vi "replace cursor - plot ref - V4.vi"(0 "plot ref IN":refnum<vi>, 1 "new X":dbl=nan, 3 "new  Y":dbl=nan, 4 "window IN":T2={"window y"=0.0021014740628288917, "center x"=44850.89441339177, "center y"=2.5658109925320947, "window x"=17480.201988350764} {"window x" format="%#9_9f"; "center y" format="%#9_9f"; "center x" format="%#9_9f"}, 5 "cursor index":i32, 6 "cursor action":T3=enum."write", 7 "label":enum16{"hide", "show x", "show y", "show (x,y)"}(ring), 9 "x-label":string, 11 "y-label":string, 12 "Color Box":u32(colorbox)=327424, 13 "cursor state":T4=enum."boring") -> (14 "plot ref OUT":refnum<vi>, 15 "read X":dbl, 18 "read Y":dbl, 19 "2Dwindow bounds out":T1={"min y"=0.0021014740628288917, "max x"=44850.89441339177, "min x"=2.5658109925320947, "max y"=17480.201988350764} {"max y" format="%#9_9f"; "min x" format="%#9_9f"; "max x" format="%#9_9f"})   [LabVIEW 2021]
uses:
  cursor sate.ctl
  cursor action.ctl
  2Dwindow-centerwin.ctl
  2Dwindow-bounds.ctl
  stack action -- control.ctl
  range multiplier action.ctl
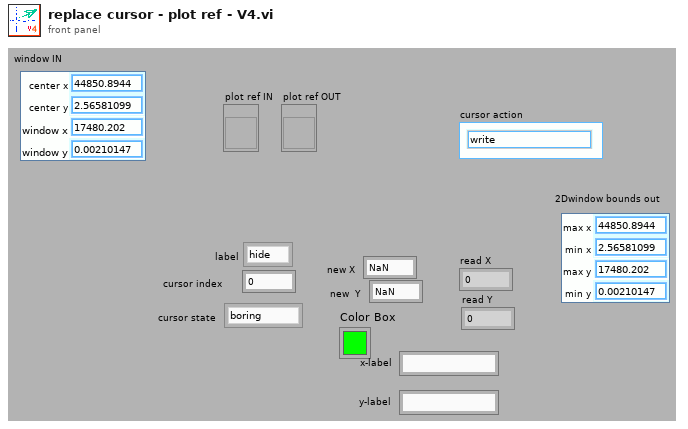
[diagram p1: front panel]
types:
  T1 = typedef "2Dwindow-bounds.ctl" = cluster{"min y":dbl, "max x":dbl, "min x":dbl, "max y":dbl}
  T2 = typedef "2Dwindow-centerwin.ctl" = cluster{"window y":dbl, "center x":dbl, "center y":dbl, "window x":dbl}
  T3 = typedef "cursor action.ctl" = enum16{"range", "read", "write", "check", "zoom out", "smart zoom out", "zoom to aspect ratio 1", "zoom to win", "zoom out 20%", "zoom in 20%", "-empty", "smart zoom out&aspect", "move range left 20%", "move range right 20%", "move range up 20%", "move range down 20%", "zoom to X win", "zoom to Y win", "zoom out X", "zoom out Y", "zoom in X", "zoom in Y", "check plot scale", "set plot color", "set Xlabel", "set Ylabel", "set cursor color", "setlength", "empty", "hide plot", "unhide plot", "checklngth", "extend +1 if short", "extend +n if short"}
  T4 = typedef "cursor sate.ctl" = enum16{"normal", "alert", "fuzzy", "interesting", "boring", "colored"}
  T5 = typedef "stack action -- control.ctl" = enum16{"push", "pop", "check", "init"}
  T6 = typedef "LVCursorListTypeDef.ctl" = cluster{"Name":string, "Color":u32, "Style":u8, "Point Style":u8, "Name Visible":bool, "Allow Drag":bool, "Cursor Mode":u32, "Plot":i32, "Index":i32, "Position":cluster{"X":dbl, "Y":dbl}, "X Scale":u32, "Y Scale":u32, "Watch Plots":i32[], "Watch All Plots":bool, "Plot Area":i32, "Label Offset":cluster{"X":dbl, "Y":dbl}}[]
  T7 = typedef "range multiplier action.ctl" = enum16{"shift", "zoom", "check"}
  T8 = cluster{"Name":string, "Color":u32, "Style":u8, "Point Style":u8, "Name Visible":bool, "Allow Drag":bool, "Cursor Mode":u32, "Plot":i32, "Index":i32, "Position":cluster{"X":dbl, "Y":dbl}, "X Scale":u32, "Y Scale":u32, "Watch Plots":i32[], "Watch All Plots":bool, "Plot Area":i32, "Label Offset":cluster{"X":dbl, "Y":dbl}}
  T9 = typedef "LVRangeTypeDef.ctl" = cluster{"Minimum":dbl, "Maximum":dbl, "Increment":dbl, "Minor Increment":dbl, "Start":dbl}
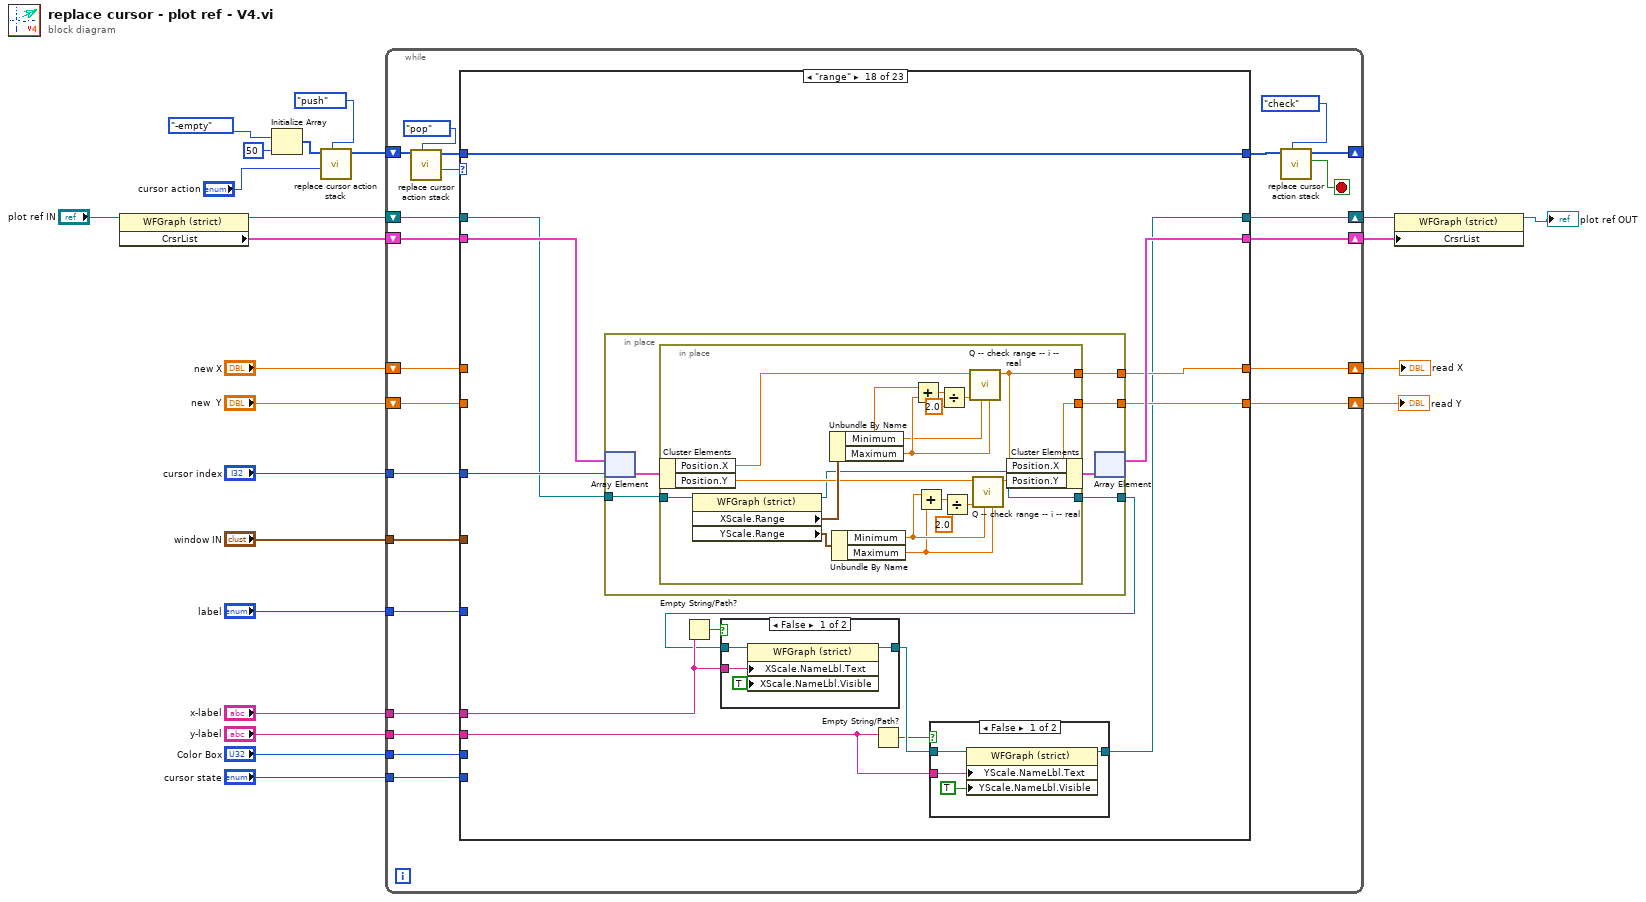
[diagram p0: block diagram]
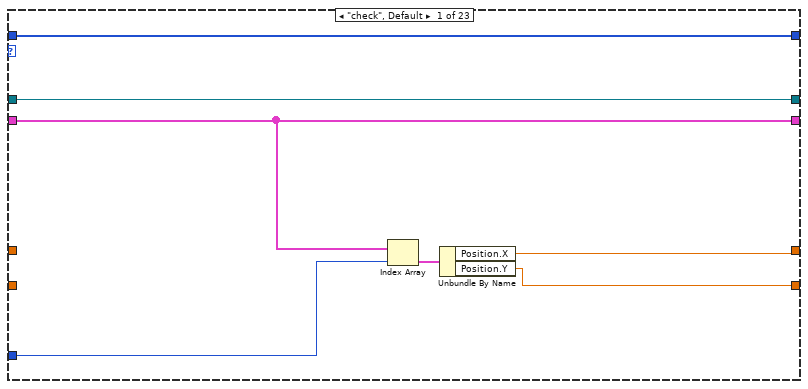
[diagram p2: hidden frame]
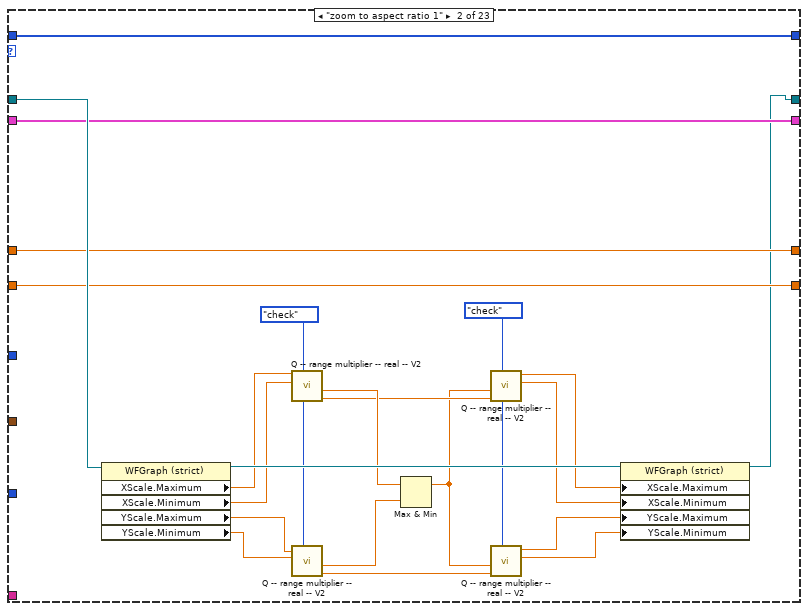
[diagram p3: hidden frame]
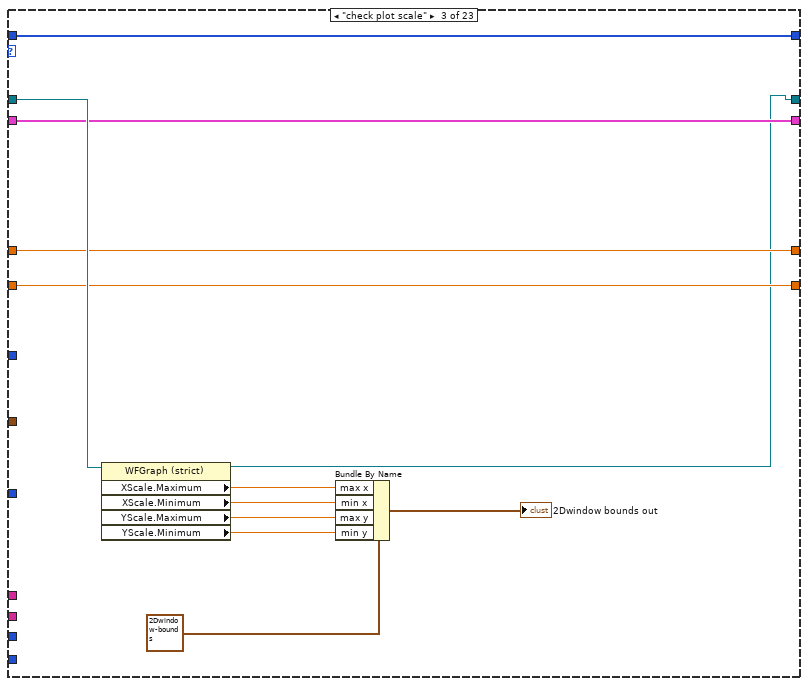
[diagram p4: hidden frame]
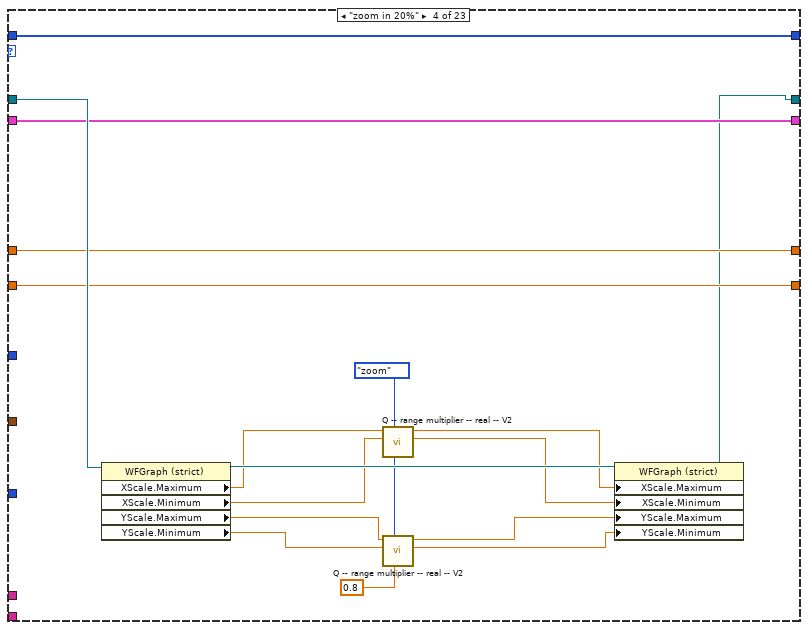
[diagram p5: hidden frame]
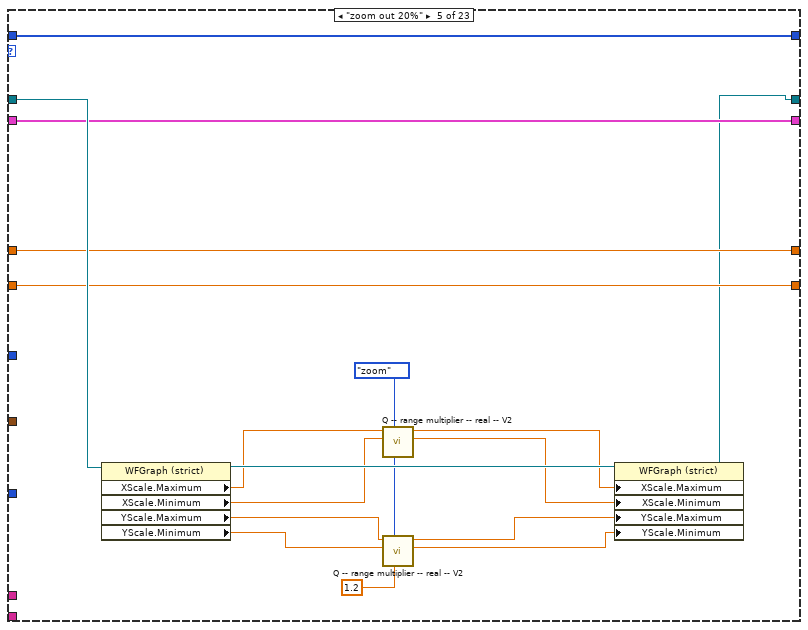
[diagram p6: hidden frame]
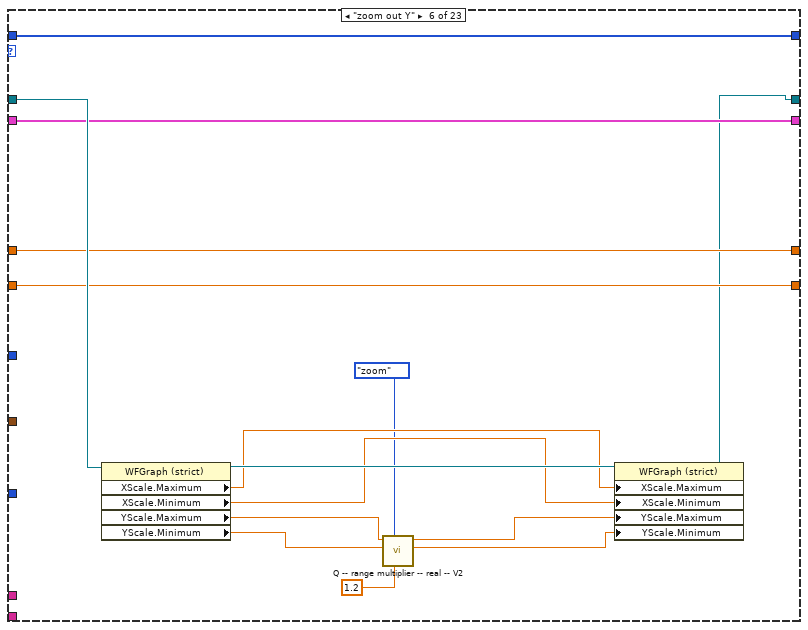
[diagram p7: hidden frame]
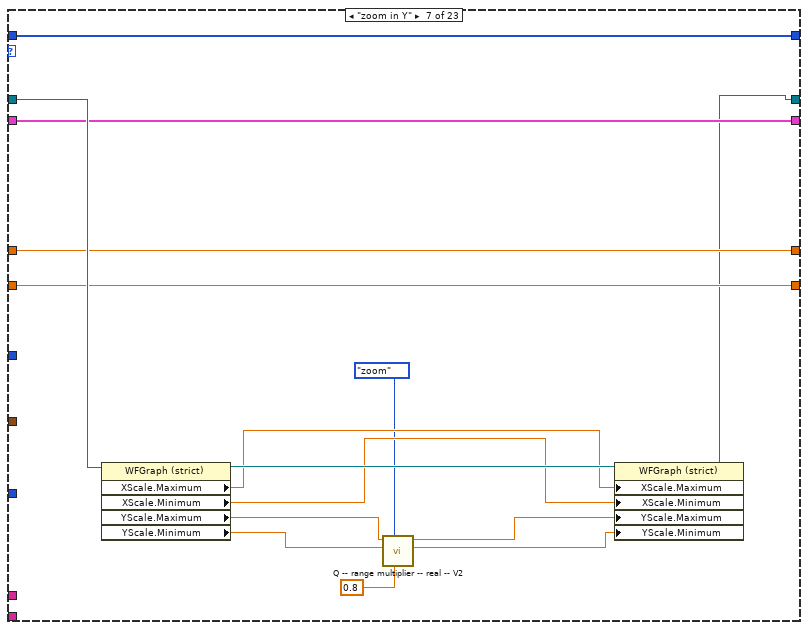
[diagram p8: hidden frame]
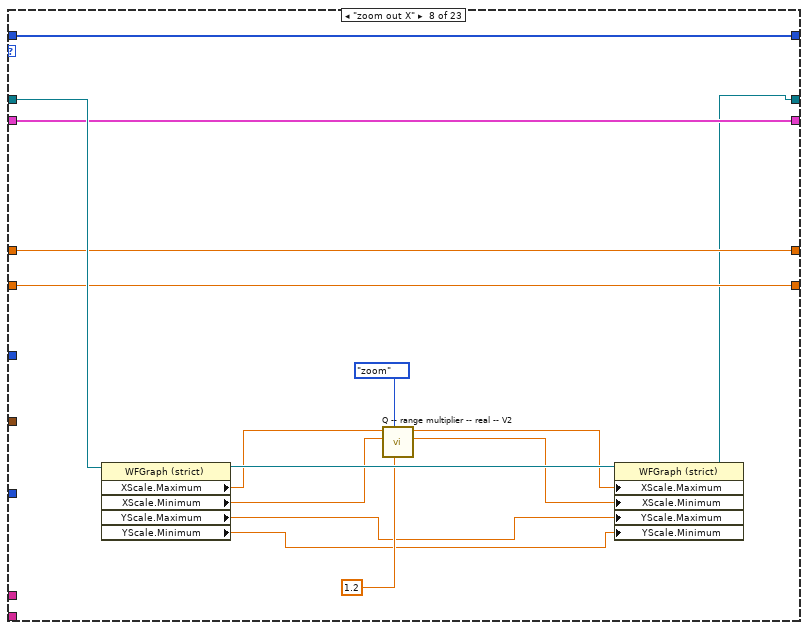
[diagram p9: hidden frame]
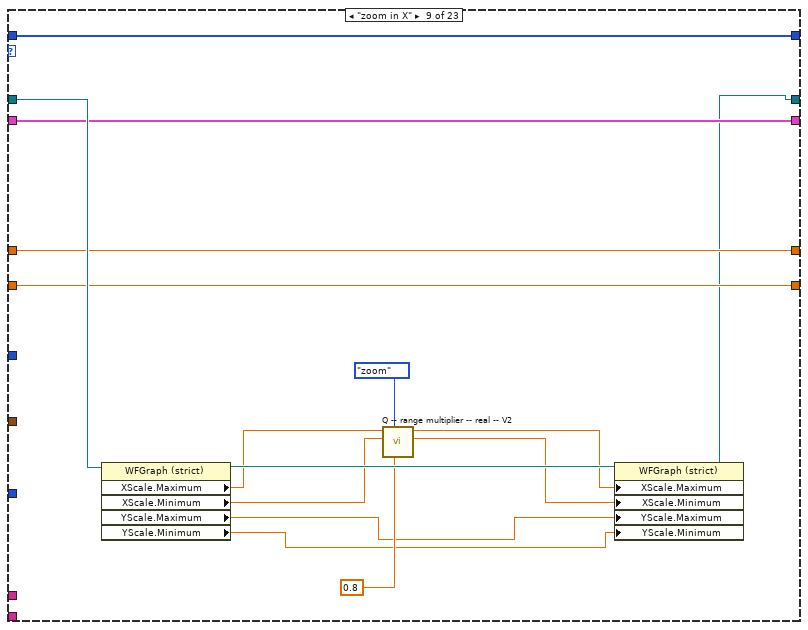
[diagram p10: hidden frame]
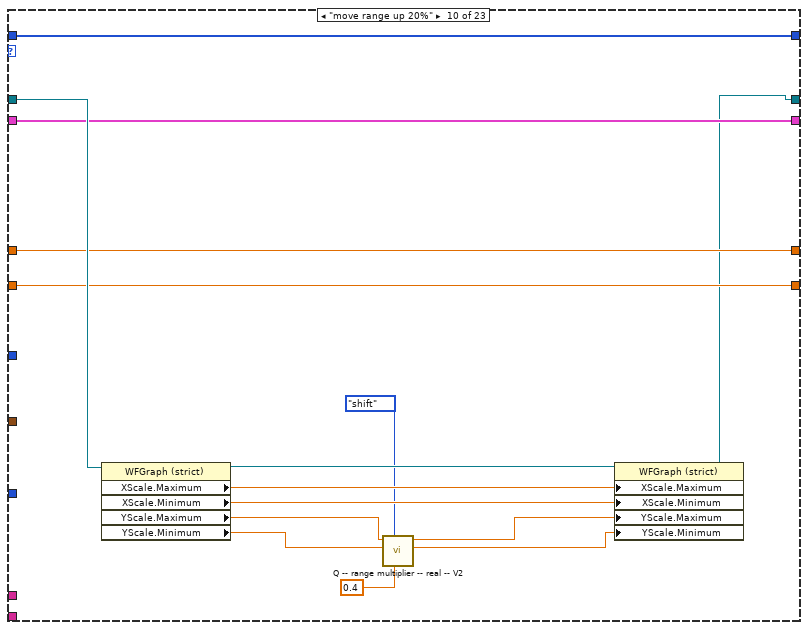
[diagram p11: hidden frame]
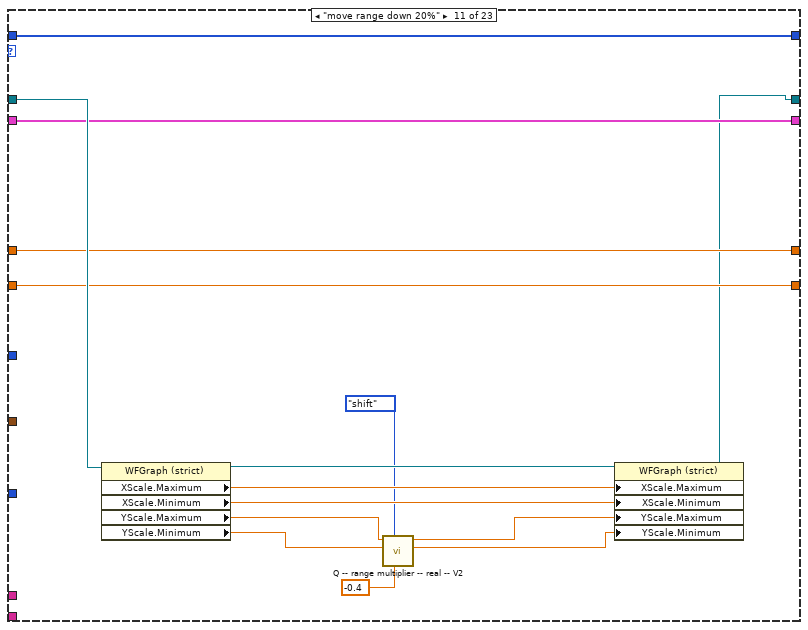
[diagram p12: hidden frame]
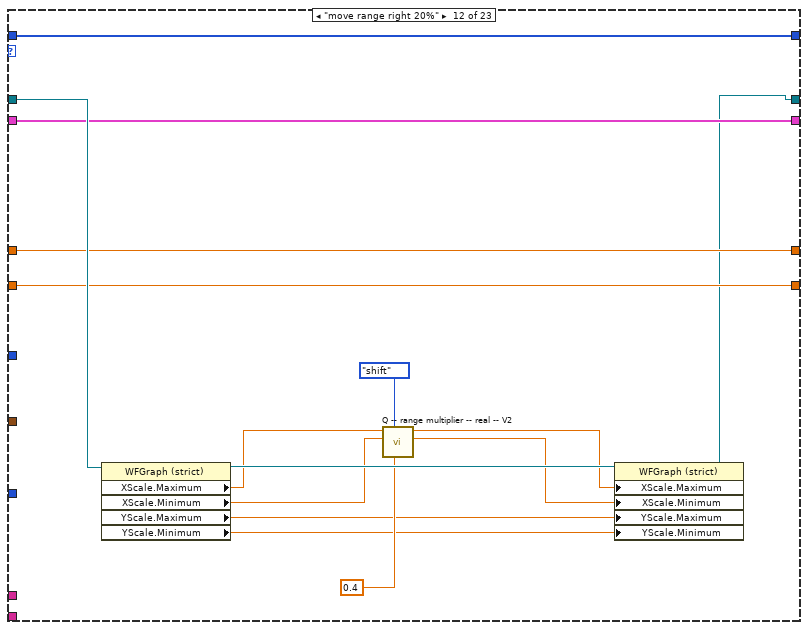
[diagram p13: hidden frame]
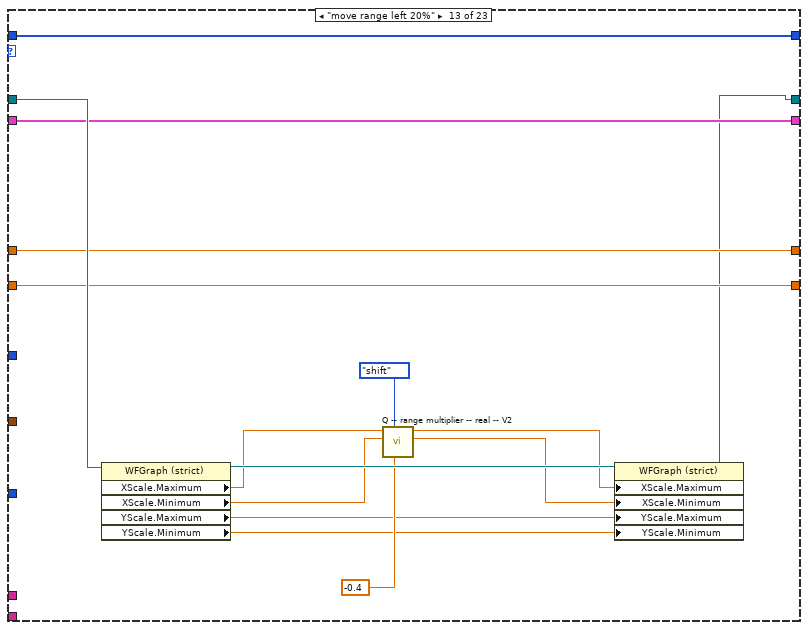
[diagram p14: hidden frame]
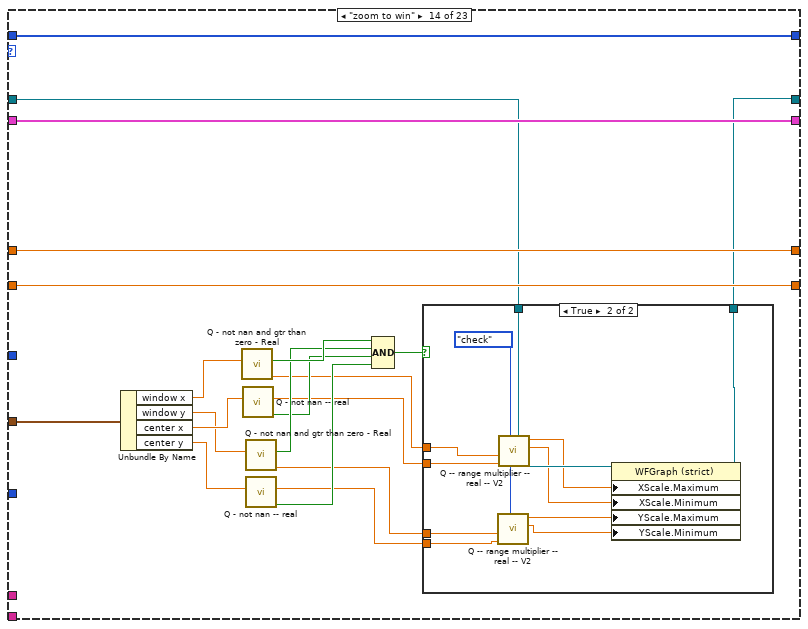
[diagram p15: hidden frame]
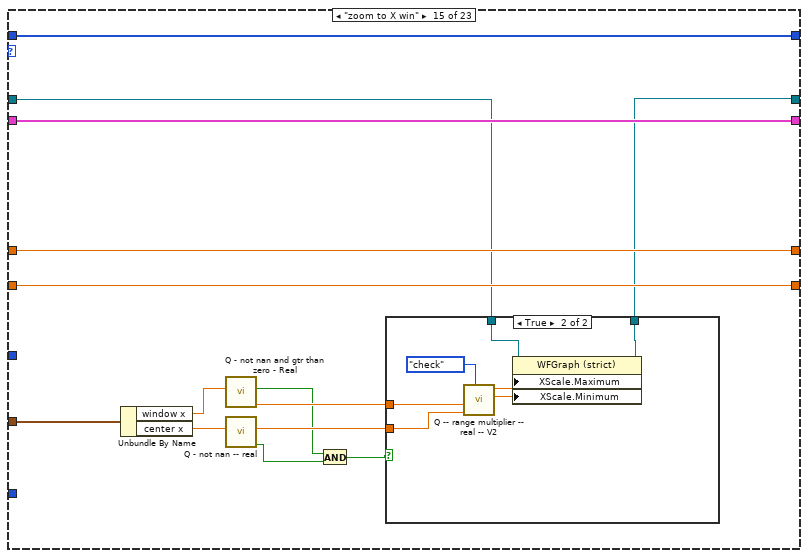
[diagram p17: hidden frame]
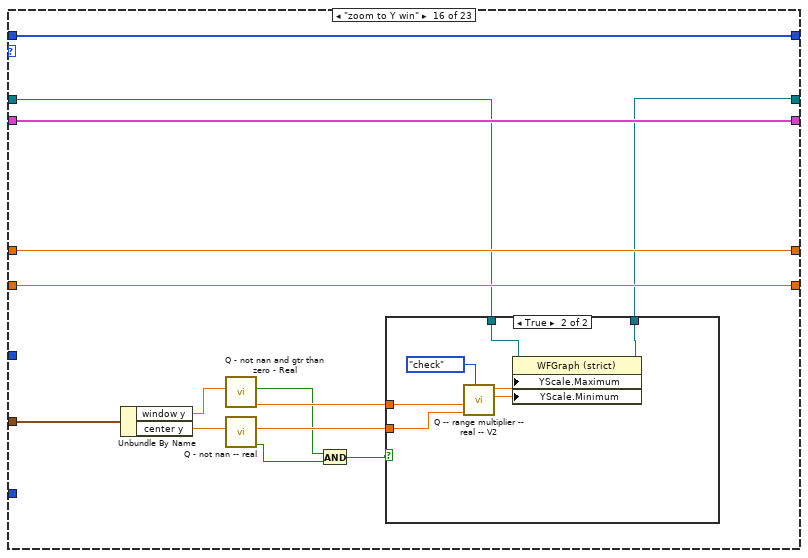
[diagram p19: hidden frame]
diagram:
  n1 = property on="Property Node" class="WFGraph (strict)"(reference="plot ref IN") -> (reference out=w15:refnum<vi>, "CrsrList"=w20:T6)  [unwired: 1 in, 1 out]
  n2 = Initialize Array(cursor_action."-empty" ("cursor action"), 50 ("dimension size")) -> (w8:T3[])
  n3 = call "replace cursor action stack.vi"("stack action"=stack_action_--_control."push", "cursor action"="cursor action", "command stack In"=w8) -> ("command stack Out"=w5:T3[])  [unwired: 6 in, 2 out]
  n4 = while {
    tunnel: "cursor index" -> [w46]
    tunnel: "label" -> [w42]
    tunnel: "Color Box" -> [w41]
    tunnel: "cursor state" -> [w40]
    tunnel: "x-label" -> [w37]
    tunnel: "y-label" -> [w36]
    tunnel: "window IN" -> [w34]
    shift-right: [w35] -> w12
    shift-left: w20 -> [w43]
    shift-right: [w39] -> w16
    shift-left: w15 -> [w38]
    shift-right: [w29] -> _
    shift-left: w5 -> [w33]
    shift-right: [w26] -> w3
    shift-left: "new  Y" -> [w45]
    shift-right: [w25] -> w4
    shift-left: "new X" -> [w44]
    stop <- w30 stop-if-true
    n5 = call "replace cursor action stack.vi"("stack action"=stack_action_--_control."pop", "command stack In"=w33) -> ("cursor action Out"=w31:T3, "command stack Out"=w27:T3[])  [unwired: 7 in, 1 out]
    n6 = case shown="\"range\"" w31 {
      tunnel: w46 -> [w51 _ _ _ _ _ _ _ _ _ _ _ _ _ _ _ _ w337 _ _ w453 w462 w507]
      tunnel: w43 -> [w52 w73 w86 w102 w119 w134 w149 w164 w179 w194 w209 w224 w239 w261 w287 w309 w318 w339 w395 w431 w451 w464 w509]
      tunnel: w45 -> [_ w71 w84 w100 w117 w132 w147 w162 w177 w192 w207 w222 w237 w259 w285 w307 w320 _ w390 w426 _ w465 w501]
      tunnel: w44 -> [_ w72 w85 w101 w118 w133 w148 w163 w178 w193 w208 w223 w238 w260 w286 w308 w321 _ w391 w427 _ w466 w502]
      tunnel: [w49 w72 w85 w101 w118 w133 w148 w163 w178 w193 w208 w223 w238 w260 w286 w308 w321 w336 w391 w427 w450 w461 w502] -> w25
      tunnel: [w48 w71 w84 w100 w117 w132 w147 w162 w177 w192 w207 w222 w237 w259 w285 w307 w320 w335 w390 w426 w449 w460 w501] -> w26
      tunnel: w42 -> [_ _ _ _ _ _ _ _ _ _ _ _ _ _ _ _ _ _ _ _ _ w459 w506]
      tunnel: w41 -> [_ _ _ _ _ _ _ _ _ _ _ _ _ _ _ _ _ _ _ _ _ w458 w505]
      tunnel: w40 -> [_ _ _ _ _ _ _ _ _ _ _ _ _ _ _ _ _ _ _ _ _ w457 _]
      tunnel: [w53 w69 w82 w98 w115 w130 w145 w160 w175 w190 w205 w220 w235 w255 w281 w303 w319 w327 w392 w428 w448 w456 w504] -> w39
      tunnel: w38 -> [w53 w74 w87 w103 w120 w135 w150 w165 w180 w195 w210 w225 w240 w257 w283 w305 w319 w334 w394 w430 w448 w456 w504]
      tunnel: w37 -> [_ _ _ _ _ _ _ _ _ _ _ _ _ _ _ _ _ w332 _ _ _ _ _]
      tunnel: w36 -> [_ _ _ _ _ _ _ _ _ _ _ _ _ _ _ _ _ w329 _ _ _ _ _]
      tunnel: [w52 w73 w86 w102 w119 w134 w149 w164 w179 w194 w209 w224 w239 w261 w287 w309 w318 w338 w395 w431 w451 w463 w508] -> w35
      tunnel: w34 -> [_ _ _ _ _ _ _ _ _ _ _ _ _ w258 w284 w306 _ _ _ _ _ _ _]
      tunnel: [w47 w70 w83 w99 w116 w131 w146 w161 w176 w191 w206 w221 w236 w256 w282 w304 w323 w326 w376 w413 w447 w455 w503] -> w28
      tunnel: w27 -> [w47 w70 w83 w99 w116 w131 w146 w161 w176 w191 w206 w221 w236 w256 w282 w304 w324 w326 w376 w413 w447 w455 w503]
      frame "check", Default {
        n7 = Index Array(array=w52, index=w51) -> (element=w50:T8)
        n8 = Unbundle By Name(w50) -> ("Position.X"=w49:dbl, "Position.Y"=w48:dbl)
      }
      frame "zoom to aspect ratio 1" {
        w58 = range_multiplier_action."check" ("rage multiplier action")
        w64 = range_multiplier_action."check" ("rage multiplier action")
        n9 = property on="Property Node" class="WFGraph (strict)"(reference=w74) -> (reference out=w75:refnum<vi>, "XScale.Maximum"=w68:dbl, "XScale.Minimum"=w67:dbl, "YScale.Maximum"=w66:dbl, "YScale.Minimum"=w65:dbl)  [unwired: 1 in, 1 out]
        n10 = call "Q -- range multiplier -- real -- V2.vi"("rage multiplier action"=w64, "lower"=w67, "upper"=w68) -> ("center OUT"=w61:dbl, "window OUT"=w63:dbl)  [unwired: 5 in, 2 out]
        n11 = call "Q -- range multiplier -- real -- V2.vi"("rage multiplier action"=w64, "lower"=w65, "upper"=w66) -> ("center OUT"=w60:dbl, "window OUT"=w62:dbl)  [unwired: 5 in, 2 out]
        n12 = Max & Min(x=w63, y=w62) -> (max(x,y)=w59:dbl)  [unwired: 1 out]
        n13 = call "Q -- range multiplier -- real -- V2.vi"("rage multiplier action"=w58, "center"=w61, "window"=w59) -> ("lower OUT"=w54:dbl, "upper OUT"=w55:dbl)  [unwired: 5 in, 2 out]
        n14 = call "Q -- range multiplier -- real -- V2.vi"("rage multiplier action"=w58, "center"=w60, "window"=w59) -> ("lower OUT"=w56:dbl, "upper OUT"=w57:dbl)  [unwired: 5 in, 2 out]
        n15 = property on="Property Node" class="WFGraph (strict)"(reference=w75, "XScale.Maximum"=w55, "XScale.Minimum"=w54, "YScale.Maximum"=w57, "YScale.Minimum"=w56) -> (reference out=w69:refnum<vi>)  [unwired: 1 in, 1 out]
      }
      frame "check plot scale" {
        n16 = property on="Property Node" class="WFGraph (strict)"(reference=w87) -> (reference out=w82:refnum<vi>, "XScale.Maximum"=w80:dbl, "XScale.Minimum"=w79:dbl, "YScale.Maximum"=w78:dbl, "YScale.Minimum"=w77:dbl)  [unwired: 1 in, 1 out]
        n17 = Bundle By Name(cluster=T1 {"min y"=0.0021014740628288917, "max x"=44850.89441339177, "min x"=2.5658109925320947, "max y"=17480.201988350764} ("2Dwindow bounds out"), "max x"=w80, "min x"=w79, "max y"=w78, "min y"=w77) -> (→"2Dwindow bounds out":T1)
      }
      frame "zoom in 20%" {
        w89 = range_multiplier_action."zoom" ("rage multiplier action")
        w88 = 0.8
        n18 = property on="Property Node" class="WFGraph (strict)"(reference=w103) -> (reference out=w104:refnum<vi>, "XScale.Maximum"=w97:dbl, "XScale.Minimum"=w96:dbl, "YScale.Maximum"=w93:dbl, "YScale.Minimum"=w92:dbl)  [unwired: 1 in, 1 out]
        n19 = call "Q -- range multiplier -- real -- V2.vi"("factor"=w88, "rage multiplier action"=w89, "lower"=w96, "upper"=w97) -> ("lower OUT"=w94:dbl, "upper OUT"=w95:dbl)  [unwired: 4 in, 2 out]
        n20 = call "Q -- range multiplier -- real -- V2.vi"("factor"=w88, "rage multiplier action"=w89, "lower"=w92, "upper"=w93) -> ("lower OUT"=w90:dbl, "upper OUT"=w91:dbl)  [unwired: 4 in, 2 out]
        n21 = property on="Property Node" class="WFGraph (strict)"(reference=w104, "XScale.Maximum"=w95, "XScale.Minimum"=w94, "YScale.Maximum"=w91, "YScale.Minimum"=w90) -> (reference out=w98:refnum<vi>)  [unwired: 1 in, 1 out]
      }
      frame "zoom out 20%" {
        w106 = range_multiplier_action."zoom" ("rage multiplier action")
        w105 = 1.2
        n22 = property on="Property Node" class="WFGraph (strict)"(reference=w120) -> (reference out=w121:refnum<vi>, "XScale.Maximum"=w114:dbl, "XScale.Minimum"=w113:dbl, "YScale.Maximum"=w110:dbl, "YScale.Minimum"=w109:dbl)  [unwired: 1 in, 1 out]
        n23 = call "Q -- range multiplier -- real -- V2.vi"("factor"=w105, "rage multiplier action"=w106, "lower"=w113, "upper"=w114) -> ("lower OUT"=w111:dbl, "upper OUT"=w112:dbl)  [unwired: 4 in, 2 out]
        n24 = call "Q -- range multiplier -- real -- V2.vi"("factor"=w105, "rage multiplier action"=w106, "lower"=w109, "upper"=w110) -> ("lower OUT"=w107:dbl, "upper OUT"=w108:dbl)  [unwired: 4 in, 2 out]
        n25 = property on="Property Node" class="WFGraph (strict)"(reference=w121, "XScale.Maximum"=w112, "XScale.Minimum"=w111, "YScale.Maximum"=w108, "YScale.Minimum"=w107) -> (reference out=w115:refnum<vi>)  [unwired: 1 in, 1 out]
      }
      frame "zoom out Y" {
        n26 = property on="Property Node" class="WFGraph (strict)"(reference=w135) -> (reference out=w136:refnum<vi>, "XScale.Maximum"=w124:dbl, "XScale.Minimum"=w123:dbl, "YScale.Maximum"=w129:dbl, "YScale.Minimum"=w128:dbl)  [unwired: 1 in, 1 out]
        n27 = call "Q -- range multiplier -- real -- V2.vi"("factor"=1.2, "rage multiplier action"=range_multiplier_action."zoom", "lower"=w128, "upper"=w129) -> ("lower OUT"=w126:dbl, "upper OUT"=w127:dbl)  [unwired: 4 in, 2 out]
        n28 = property on="Property Node" class="WFGraph (strict)"(reference=w136, "XScale.Maximum"=w124, "XScale.Minimum"=w123, "YScale.Maximum"=w127, "YScale.Minimum"=w126) -> (reference out=w130:refnum<vi>)  [unwired: 1 in, 1 out]
      }
      frame "zoom in Y" {
        n29 = property on="Property Node" class="WFGraph (strict)"(reference=w150) -> (reference out=w151:refnum<vi>, "XScale.Maximum"=w139:dbl, "XScale.Minimum"=w138:dbl, "YScale.Maximum"=w144:dbl, "YScale.Minimum"=w143:dbl)  [unwired: 1 in, 1 out]
        n30 = call "Q -- range multiplier -- real -- V2.vi"("factor"=0.8, "rage multiplier action"=range_multiplier_action."zoom", "lower"=w143, "upper"=w144) -> ("lower OUT"=w141:dbl, "upper OUT"=w142:dbl)  [unwired: 4 in, 2 out]
        n31 = property on="Property Node" class="WFGraph (strict)"(reference=w151, "XScale.Maximum"=w139, "XScale.Minimum"=w138, "YScale.Maximum"=w142, "YScale.Minimum"=w141) -> (reference out=w145:refnum<vi>)  [unwired: 1 in, 1 out]
      }
      frame "zoom out X" {
        n32 = property on="Property Node" class="WFGraph (strict)"(reference=w165) -> (reference out=w166:refnum<vi>, "XScale.Maximum"=w159:dbl, "XScale.Minimum"=w158:dbl, "YScale.Maximum"=w153:dbl, "YScale.Minimum"=w152:dbl)  [unwired: 1 in, 1 out]
        n33 = call "Q -- range multiplier -- real -- V2.vi"("factor"=1.2, "rage multiplier action"=range_multiplier_action."zoom", "lower"=w158, "upper"=w159) -> ("lower OUT"=w156:dbl, "upper OUT"=w157:dbl)  [unwired: 4 in, 2 out]
        n34 = property on="Property Node" class="WFGraph (strict)"(reference=w166, "XScale.Maximum"=w157, "XScale.Minimum"=w156, "YScale.Maximum"=w153, "YScale.Minimum"=w152) -> (reference out=w160:refnum<vi>)  [unwired: 1 in, 1 out]
      }
      frame "zoom in X" {
        n35 = property on="Property Node" class="WFGraph (strict)"(reference=w180) -> (reference out=w181:refnum<vi>, "XScale.Maximum"=w174:dbl, "XScale.Minimum"=w173:dbl, "YScale.Maximum"=w168:dbl, "YScale.Minimum"=w167:dbl)  [unwired: 1 in, 1 out]
        n36 = call "Q -- range multiplier -- real -- V2.vi"("factor"=0.8, "rage multiplier action"=range_multiplier_action."zoom", "lower"=w173, "upper"=w174) -> ("lower OUT"=w171:dbl, "upper OUT"=w172:dbl)  [unwired: 4 in, 2 out]
        n37 = property on="Property Node" class="WFGraph (strict)"(reference=w181, "XScale.Maximum"=w172, "XScale.Minimum"=w171, "YScale.Maximum"=w168, "YScale.Minimum"=w167) -> (reference out=w175:refnum<vi>)  [unwired: 1 in, 1 out]
      }
      frame "move range up 20%" {
        n38 = property on="Property Node" class="WFGraph (strict)"(reference=w195) -> (reference out=w196:refnum<vi>, "XScale.Maximum"=w183:dbl, "XScale.Minimum"=w184:dbl, "YScale.Maximum"=w189:dbl, "YScale.Minimum"=w188:dbl)  [unwired: 1 in, 1 out]
        n39 = call "Q -- range multiplier -- real -- V2.vi"("factor"=0.4, "rage multiplier action"=range_multiplier_action."shift", "lower"=w188, "upper"=w189) -> ("lower OUT"=w186:dbl, "upper OUT"=w187:dbl)  [unwired: 4 in, 2 out]
        n40 = property on="Property Node" class="WFGraph (strict)"(reference=w196, "XScale.Maximum"=w183, "XScale.Minimum"=w184, "YScale.Maximum"=w187, "YScale.Minimum"=w186) -> (reference out=w190:refnum<vi>)  [unwired: 1 in, 1 out]
      }
      frame "move range down 20%" {
        n41 = property on="Property Node" class="WFGraph (strict)"(reference=w210) -> (reference out=w211:refnum<vi>, "XScale.Maximum"=w198:dbl, "XScale.Minimum"=w199:dbl, "YScale.Maximum"=w204:dbl, "YScale.Minimum"=w203:dbl)  [unwired: 1 in, 1 out]
        n42 = call "Q -- range multiplier -- real -- V2.vi"("factor"=-0.4, "rage multiplier action"=range_multiplier_action."shift", "lower"=w203, "upper"=w204) -> ("lower OUT"=w201:dbl, "upper OUT"=w202:dbl)  [unwired: 4 in, 2 out]
        n43 = property on="Property Node" class="WFGraph (strict)"(reference=w211, "XScale.Maximum"=w198, "XScale.Minimum"=w199, "YScale.Maximum"=w202, "YScale.Minimum"=w201) -> (reference out=w205:refnum<vi>)  [unwired: 1 in, 1 out]
      }
      frame "move range right 20%" {
        n44 = property on="Property Node" class="WFGraph (strict)"(reference=w225) -> (reference out=w226:refnum<vi>, "XScale.Maximum"=w219:dbl, "XScale.Minimum"=w218:dbl, "YScale.Maximum"=w213:dbl, "YScale.Minimum"=w212:dbl)  [unwired: 1 in, 1 out]
        n45 = call "Q -- range multiplier -- real -- V2.vi"("factor"=0.4, "rage multiplier action"=range_multiplier_action."shift", "lower"=w218, "upper"=w219) -> ("lower OUT"=w216:dbl, "upper OUT"=w217:dbl)  [unwired: 4 in, 2 out]
        n46 = property on="Property Node" class="WFGraph (strict)"(reference=w226, "XScale.Maximum"=w217, "XScale.Minimum"=w216, "YScale.Maximum"=w213, "YScale.Minimum"=w212) -> (reference out=w220:refnum<vi>)  [unwired: 1 in, 1 out]
      }
      frame "move range left 20%" {
        n47 = property on="Property Node" class="WFGraph (strict)"(reference=w240) -> (reference out=w241:refnum<vi>, "XScale.Maximum"=w234:dbl, "XScale.Minimum"=w233:dbl, "YScale.Maximum"=w228:dbl, "YScale.Minimum"=w227:dbl)  [unwired: 1 in, 1 out]
        n48 = call "Q -- range multiplier -- real -- V2.vi"("factor"=-0.4, "rage multiplier action"=range_multiplier_action."shift", "lower"=w233, "upper"=w234) -> ("lower OUT"=w231:dbl, "upper OUT"=w232:dbl)  [unwired: 4 in, 2 out]
        n49 = property on="Property Node" class="WFGraph (strict)"(reference=w241, "XScale.Maximum"=w232, "XScale.Minimum"=w231, "YScale.Maximum"=w228, "YScale.Minimum"=w227) -> (reference out=w235:refnum<vi>)  [unwired: 1 in, 1 out]
      }
      frame "zoom to win" {
        n50 = Unbundle By Name(w258) -> ("window x"=w254:dbl, "window y"=w251:dbl, "center x"=w252:dbl, "center y"=w253:dbl)
        n51 = call "Q - not nan and gtr than zero - Real.vi"("Numeric"=w254) -> ("number out"=w245:dbl, "answer"=w250:bool)  [unwired: 9 in]
        n52 = call "Q - not nan -- real.vi"("Numeric"=w252) -> ("Boolean"=w248:bool, "out"=w244:dbl)  [unwired: 9 in]
        n53 = call "Q - not nan and gtr than zero - Real.vi"("Numeric"=w251) -> ("number out"=w243:dbl, "answer"=w249:bool)  [unwired: 9 in]
        n54 = call "Q - not nan -- real.vi"("Numeric"=w253) -> ("Boolean"=w247:bool, "out"=w242:dbl)  [unwired: 9 in]
        n55 = Compound Arithmetic op=AND(w250, w249, w248, w247) -> (w246:bool)
        n56 = case shown="True" w246 {
          tunnel: w257 -> [w262 w273]
          tunnel: [w262 w272] -> w255
          tunnel: w245 -> [_ w266]
          tunnel: w244 -> [_ w265]
          tunnel: w243 -> [_ w264]
          tunnel: w242 -> [_ w263]
          frame False {
          }
          frame True {
            w271 = range_multiplier_action."check" ("rage multiplier action")
            n57 = call "Q -- range multiplier -- real -- V2.vi"("rage multiplier action"=w271, "center"=w263, "window"=w264) -> ("lower OUT"=w270:dbl, "upper OUT"=w267:dbl)  [unwired: 5 in, 2 out]
            n58 = call "Q -- range multiplier -- real -- V2.vi"("rage multiplier action"=w271, "center"=w265, "window"=w266) -> ("lower OUT"=w269:dbl, "upper OUT"=w268:dbl)  [unwired: 5 in, 2 out]
            n59 = property on="Property Node" class="WFGraph (strict)"(reference=w273, "XScale.Maximum"=w268, "XScale.Minimum"=w269, "YScale.Maximum"=w267, "YScale.Minimum"=w270) -> (reference out=w272:refnum<vi>)  [unwired: 1 in, 1 out]
          }
        }
      }
      frame "zoom to X win" {
        n60 = Unbundle By Name(w284) -> ("window x"=w280:dbl, "center x"=w278:dbl)
        n61 = call "Q - not nan and gtr than zero - Real.vi"("Numeric"=w280) -> ("number out"=w279:dbl, "answer"=w276:bool)  [unwired: 9 in]
        n62 = call "Q - not nan -- real.vi"("Numeric"=w278) -> ("Boolean"=w275:bool, "out"=w277:dbl)  [unwired: 9 in]
        n63 = And(x=w276, y=w275) -> (x .and. y?=w274:bool)
        n64 = case shown="True" w274 {
          tunnel: w283 -> [w288 w295]
          tunnel: [w288 w294] -> w281
          tunnel: w279 -> [_ w290]
          tunnel: w277 -> [_ w289]
          frame False {
          }
          frame True {
            n65 = call "Q -- range multiplier -- real -- V2.vi"("rage multiplier action"=range_multiplier_action."check", "center"=w289, "window"=w290) -> ("lower OUT"=w292:dbl, "upper OUT"=w291:dbl)  [unwired: 5 in, 2 out]
            n66 = property on="Property Node" class="WFGraph (strict)"(reference=w295, "XScale.Maximum"=w291, "XScale.Minimum"=w292) -> (reference out=w294:refnum<vi>)  [unwired: 1 in, 1 out]
          }
        }
      }
      frame "zoom to Y win" {
        n67 = Unbundle By Name(w306) -> ("window y"=w302:dbl, "center y"=w300:dbl)
        n68 = call "Q - not nan and gtr than zero - Real.vi"("Numeric"=w302) -> ("number out"=w301:dbl, "answer"=w298:bool)  [unwired: 9 in]
        n69 = call "Q - not nan -- real.vi"("Numeric"=w300) -> ("Boolean"=w297:bool, "out"=w299:dbl)  [unwired: 9 in]
        n70 = And(x=w298, y=w297) -> (x .and. y?=w296:bool)
        n71 = case shown="True" w296 {
          tunnel: w305 -> [w310 w317]
          tunnel: [w310 w316] -> w303
          tunnel: w301 -> [_ w312]
          tunnel: w299 -> [_ w311]
          frame False {
          }
          frame True {
            n72 = call "Q -- range multiplier -- real -- V2.vi"("rage multiplier action"=range_multiplier_action."check", "center"=w311, "window"=w312) -> ("lower OUT"=w314:dbl, "upper OUT"=w313:dbl)  [unwired: 5 in, 2 out]
            n73 = property on="Property Node" class="WFGraph (strict)"(reference=w317, "YScale.Maximum"=w313, "YScale.Minimum"=w314) -> (reference out=w316:refnum<vi>)  [unwired: 1 in, 1 out]
          }
        }
      }
      frame "smart zoom out&aspect" {
        w322 = T3[] [enum."smart zoom out", enum."zoom to aspect ratio 1"] items=["range", "read", "write", "check", "zoom out", "smart zoom out", "zoom to aspect ratio 1", "zoom to win", "zoom out 20%", "zoom in 20%", "-empty", "smart zoom out&aspect", "move range left 20%", "move range right 20%", "move range up 20%", "move range down 20%", "zoom to X win", "zoom to Y win", "zoom out X", "zoom out Y", "zoom in X", "zoom in Y", "check plot scale", "set plot color", "set Xlabel", "set Ylabel", "set cursor color", "setlength", "empty", "hide plot", "unhide plot", "checklngth", "extend +1 if short", "extend +n if short"] ("action list I")
        n74 = call "replace cursor action stack.vi"("stack action"=stack_action_--_control."push", "action list I"=w322, "command stack In"=w324) -> ("command stack Out"=w323:T3[])  [unwired: 6 in, 2 out]
      }
      frame "range" {
        n75 = in-place {
          in-place-border: w334 -> [w353]
          in-place-border: [w352] -> w336
          in-place-border: [w351] -> w335
          in-place-border: [w350] -> w328
          n76 = in-place-array #1(w339, w337) -> (w355:T8)
          n77 = in-place {
            in-place-border: w353 -> [w361]
            in-place-border: [w358] -> w352
            in-place-border: [w357] -> w351
            in-place-border: [w356] -> w350
            n78 = in-place-cluster #2(w355) -> ("Position.X"=w360:dbl, "Position.Y"=w359:dbl)
            n79 = property on="Property Node" class="WFGraph (strict)"(reference=w361) -> (reference out=w356:refnum<vi>, "XScale.Range"=w362:T9, "YScale.Range"=w363:T9)  [unwired: 1 in, 1 out]
            n80 = Unbundle By Name(w362) -> ("Minimum"=w364:dbl, "Maximum"=w365:dbl)
            n81 = Unbundle By Name(w363) -> ("Minimum"=w373:dbl, "Maximum"=w372:dbl)
            n82 = Add(x=w364, y=w365) -> (x+y=w366:dbl)
            n83 = Add(x=w373, y=w372) -> (x+y=w369:dbl)
            n84 = Divide(x=w366, y=2.0) -> (x/y=w368:dbl)
            n85 = Divide(x=w369, y=2.0) -> (x/y=w371:dbl)
            n86 = call "Q -- check range -- i -- real.vi"("upper"=w365, "lower"=w364, "default"=w368, "number"=w360) -> ("number in range"=w358:dbl)  [unwired: 5 in, 2 out]
            n87 = call "Q -- check range -- i -- real.vi"("upper"=w372, "lower"=w373, "default"=w371, "number"=w359) -> ("number in range"=w357:dbl)  [unwired: 5 in, 2 out]
            n88 = in-place-cluster #2("Position.X"=w358, "Position.Y"=w357) -> (w354:T8)
          }
          n89 = in-place-array #1(w354) -> (w338:T6)  [unwired: 1 out]
        }
        n90 = Empty String/Path?(string/path=w332) -> (empty?=w333:bool)
        n91 = case shown="False" w333 {
          tunnel: w328 -> [w348 w349]
          tunnel: w332 -> [w347 _]
          tunnel: [w346 w349] -> w331
          frame False {
            n92 = property on="Property Node" class="WFGraph (strict)"(reference=w348, "XScale.NameLbl.Text"=w347, "XScale.NameLbl.Visible"=TRUE ("X Scale.Name Label.Visible")) -> (reference out=w346:refnum<vi>)  [unwired: 1 in, 1 out]
          }
          frame True {
          }
        }
        n93 = Empty String/Path?(string/path=w329) -> (empty?=w330:bool)
        n94 = case shown="False" w330 {
          tunnel: w331 -> [w343 w344]
          tunnel: w329 -> [w342 _]
          tunnel: [w341 w344] -> w327
          frame False {
            n95 = property on="Property Node" class="WFGraph (strict)"(reference=w343, "YScale.NameLbl.Text"=w342, "YScale.NameLbl.Visible"=TRUE ("X Scale.Name Label.Visible")) -> (reference out=w341:refnum<vi>)  [unwired: 1 in, 1 out]
          }
          frame True {
          }
        }
      }
      frame "zoom out" {
        w375 = range_multiplier_action."zoom" ("rage multiplier action")
        w377 = 1.3 ("factor")
        n96 = property on="Property Node" class="WFGraph (strict)"(reference=w394) -> (reference out=w393:refnum<vi>, "Value"=w389:cluster{"f0":dbl, "df":dbl, "magnitude":dbl[]}[])  [unwired: 1 in, 1 out]
        n97 = for {
          tunnel: w389 -> [w398] mode=indexing
          tunnel: [w402] -> w385 mode=indexing
          tunnel: [w403] -> w386 mode=indexing
          tunnel: [w404] -> w387 mode=indexing
          tunnel: [w405] -> w388 mode=indexing
          n98 = Unbundle(w398) -> ("f0"=w400:dbl, "df"=w399:dbl, "magnitude"=w401:dbl[])
          n99 = for {
            tunnel: w401 -> [w409] mode=indexing
            tunnel: [w409] -> w396 mode=indexing
            shift-right: [w407] -> _
            shift-left: w400 -> [w406]
            tunnel: w399 -> [w408]
            tunnel: [w406] -> w397 mode=indexing
            n100 = Add(x=w408, y=w406) -> (x+y=w407:dbl)
          }
          n101 = Array Max & Min(array=w397) -> (max value=w403:dbl, min value=w402:dbl)  [unwired: 2 out]
          n102 = Array Max & Min(array=w396) -> (max value=w405:dbl, min value=w404:dbl)  [unwired: 2 out]
        }
        n103 = Array Max & Min(array=w388) -> (max value=w380:dbl)  [unwired: 3 out]
        n104 = Array Max & Min(array=w387) -> (min value=w379:dbl)  [unwired: 3 out]
        n105 = Array Max & Min(array=w386) -> (max value=w378:dbl)  [unwired: 3 out]
        n106 = Array Max & Min(array=w385) -> (min value=w374:dbl)  [unwired: 3 out]
        n107 = call "Q -- range multiplier -- real -- V2.vi"("factor"=w377, "rage multiplier action"=w375, "lower"=w379, "upper"=w380) -> ("lower OUT"=w381:dbl, "upper OUT"=w382:dbl)  [unwired: 4 in, 2 out]
        n108 = call "Q -- range multiplier -- real -- V2.vi"("factor"=w377, "rage multiplier action"=w375, "lower"=w374, "upper"=w378) -> ("lower OUT"=w383:dbl, "upper OUT"=w384:dbl)  [unwired: 4 in, 2 out]
        n109 = property on="Property Node" class="WFGraph (strict)"(reference=w393, "YScale.Maximum"=w382, "YScale.Minimum"=w381, "XScale.Maximum"=w384, "XScale.Minimum"=w383) -> (reference out=w392:refnum<vi>)  [unwired: 1 in, 1 out]
      }
      frame "smart zoom out" {
        w412 = range_multiplier_action."zoom" ("rage multiplier action")
        w414 = 1.2 ("factor")
        n110 = property on="Property Node" class="WFGraph (strict)"(reference=w430) -> (reference out=w429:refnum<vi>, "Value"=w410:cluster{"f0":dbl, "df":dbl, "magnitude":dbl[]}[])  [unwired: 1 in, 1 out]
        n111 = for {
          tunnel: [w440] -> w419 mode=indexing
          tunnel: [w441] -> w417 mode=indexing
          tunnel: [w439] -> w416 mode=indexing
          tunnel: [w442] -> w421 mode=indexing
          tunnel: w410 -> [w437] mode=indexing
          w438 = 0.01 ("median range")
          n112 = Unbundle(w437) -> ("f0"=w434:dbl, "df"=w433:dbl, "magnitude"=w436:dbl[])
          n113 = for {
            tunnel: w436 -> [w446] mode=indexing
            tunnel: [w446] -> w435 mode=indexing
            shift-right: [w444] -> _
            shift-left: w434 -> [w443]
            tunnel: w433 -> [w445]
            tunnel: [w443] -> w432 mode=indexing
            n114 = Add(x=w445, y=w443) -> (x+y=w444:dbl)
          }
          n115 = call "array - smart min max.vi"("median range"=w438, "x"=w435) -> ("min"=w440:dbl, "max"=w441:dbl)  [unwired: 8 in]
          n116 = call "array - smart min max.vi"("median range"=w438, "x"=w432) -> ("min"=w439:dbl, "max"=w442:dbl)  [unwired: 8 in]
        }
        n117 = Array Max & Min(array=w421) -> (max value=w420:dbl)  [unwired: 3 out]
        n118 = Array Max & Min(array=w416) -> (min value=w415:dbl)  [unwired: 3 out]
        n119 = Array Max & Min(array=w417) -> (max value=w411:dbl)  [unwired: 3 out]
        n120 = Array Max & Min(array=w419) -> (min value=w418:dbl)  [unwired: 3 out]
        n121 = call "Q -- range multiplier -- real -- V2.vi"("factor"=w414, "rage multiplier action"=w412, "lower"=w415, "upper"=w420) -> ("lower OUT"=w422:dbl, "upper OUT"=w423:dbl)  [unwired: 4 in, 2 out]
        n122 = call "Q -- range multiplier -- real -- V2.vi"("factor"=w414, "rage multiplier action"=w412, "lower"=w418, "upper"=w411) -> ("lower OUT"=w424:dbl, "upper OUT"=w425:dbl)  [unwired: 4 in, 2 out]
        n123 = property on="Property Node" class="WFGraph (strict)"(reference=w429, "XScale.Maximum"=w423, "XScale.Minimum"=w422, "YScale.Maximum"=w425, "YScale.Minimum"=w424) -> (reference out=w428:refnum<vi>)  [unwired: 1 in, 1 out]
      }
      frame "read" {
        n124 = Index Array(array=w451, index=w453) -> (element=w454:T8)
        n125 = Unbundle By Name(w454) -> ("Position"=w452:cluster{"X":dbl, "Y":dbl})
        n126 = Unbundle By Name(w452) -> ("X"=w450:dbl, "Y"=w449:dbl)
      }
      frame "write" {
        n127 = in-place {
          in-place-border: w466 -> [w469]
          in-place-border: w465 -> [w472]
          in-place-border: [w468] -> w461
          in-place-border: [w470] -> w460
          in-place-border: w459 -> [w478]
          in-place-border: w458 -> [w475]
          in-place-border: w457 -> [w476]
          w479 = 0.4 ("Label Offset.X")
          n128 = in-place-array #3(w464, w462) -> (w482:T8)
          n129 = Unbundle By Name(w482) -> ("Color"=w473:u32, "Position.X"=w467:dbl, "Position.Y"=w471:dbl)
          n130 = call "Q - not nan -- real.vi"("default"=w471, "Numeric"=w472) -> ("out"=w470:dbl)  [unwired: 8 in, 1 out]
          n131 = call "Q - not nan -- real.vi"("default"=w467, "Numeric"=w469) -> ("out"=w468:dbl)  [unwired: 8 in, 1 out]
          n132 = case shown="\"show x\"" w478 {
            tunnel: w468 -> [_ w491 _ w497]
            tunnel: ["" ("format string") w490 w494 w500] -> w481
            tunnel: [FALSE ("Name Visible") TRUE ("Name Visible") TRUE ("Name Visible") TRUE ("Name Visible")] -> w477
            tunnel: w470 -> [_ _ w493 w496]
            frame "hide", Default {
            }
            frame "show x" {
              n133 = Number To Fractional String(number=w491, precision (6)=i16 2) -> (F-format string=w490:string)  [unwired: 2 in]
            }
            frame "show y" {
              n134 = Number To Fractional String(number=w493, precision (6)=i16 2) -> (F-format string=w494:string)  [unwired: 2 in]
            }
            frame "show (x,y)" {
              n135 = Format Into String(format string="(%4f\\n%4f)", w497, w496) -> (resulting string=w500:string)  [unwired: 2 in, 1 out]
            }
          }
          n136 = case shown="\"boring\", Default" w476 {
            tunnel: [w483 u32 327424 ("Color Box") w485] -> w474
            tunnel: w475 -> [_ _ w485]
            tunnel: w473 -> [w483 _ _]
            frame "boring", Default {
            }
            frame "interesting" {
            }
            frame "colored" {
            }
          }
          n137 = Bundle By Name(cluster=w482, "Position.X"=w468, "Position.Y"=w470, "Name"=w481, "Name Visible"=w477, "Label Offset.X"=w479, "Label Offset.Y"=w479, "Color"=w474) -> (w480:T8)
          n138 = in-place-array #3(w480) -> (w463:T6)  [unwired: 1 out]
        }
      }
      frame "set cursor color" {
        n139 = in-place {
          in-place-border: w506 -> [_]
          in-place-border: w505 -> [w510]
          n140 = in-place-array #4(w509, w507) -> (w512:T8)
          n141 = Bundle By Name(cluster=w512, "Color"=w510) -> (w511:T8)
          n142 = in-place-array #4(w511) -> (w508:T6)  [unwired: 1 out]
        }
      }
    }
    n143 = call "replace cursor action stack.vi"("stack action"=stack_action_--_control."check", "command stack In"=w28) -> ("stack is empty ?"=w30:bool, "command stack Out"=w29:T3[])  [unwired: 7 in, 1 out]
  }
  "read X" <- w4
  "read Y" <- w3
  n144 = property on="Property Node" class="WFGraph (strict)"(reference=w16, "CrsrList"=w12) -> (reference out=→"plot ref OUT":refnum<vi>)  [unwired: 1 in, 1 out]
